vi "Read N.vi"(8 "error in (no error)":errorcluster, 11 "SP in":refnum<class "Save messages PGserver.lvclass">) -> (0 "error out":errorcluster, 2 "N":i32, 3 "SP out":refnum<class "Save messages PGserver.lvclass">)   [LabVIEW 2019, in "Save messages PGserver.lvclass"]
uses:
  Save messages PGserver.lvclass
  Save messages PGserver.lvclass/Save messages PGserver.ctl
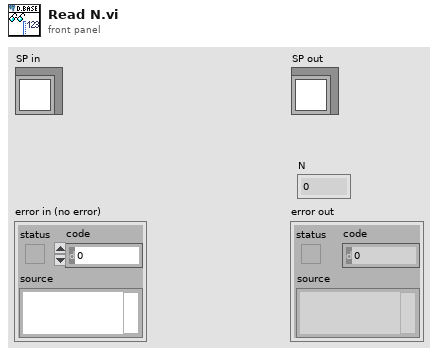
[diagram p1: front panel]
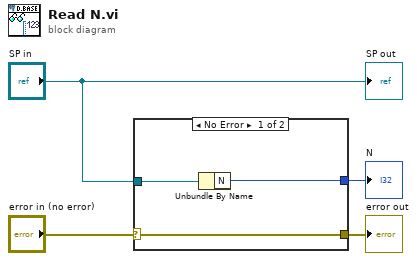
[diagram p0: block diagram]
diagram:
  n1 = case shown="No Error" "error in (no error)" {
    selector: "error in (no error)" -> [w7 w8]
    tunnel: [w7 w8] -> w3
    tunnel: "SP in" -> [w5 _]
    tunnel: [w6 _] -> w2
    frame No Error {
      n2 = Unbundle By Name(w5) -> ("N"=w6:i32)
    }
    frame Error {
    }
  }
  "error out" <- w3
  "N" <- w2
  "SP out" <- "SP in"
